vi "Decorate.vi"(10 "Queue":refnum<class "Queue.lvclass">, 11 "TEMPLATE Queue in":refnum<class "TEMPLATE Queue.lvclass">) -> (3 "TEMPLATE Queue out":refnum<class "TEMPLATE Queue.lvclass">)   [LabVIEW 2021, in "_Template.lvlib" / "Templates.lvlib" / "TEMPLATE Queue.lvlib" / "TEMPLATE Queue.lvclass"]
uses:
  TEMPLATE Queue.lvclass
  <vilib>/Nathan Davis/jettl/jettl/Queue/Queue.lvclass
  TEMPLATE Queue.lvclass/TEMPLATE Queue.ctl
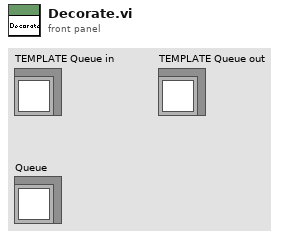
[diagram p1: front panel]
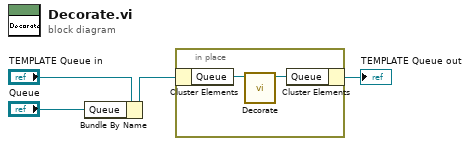
[diagram p0: block diagram]
diagram:
  n1 = Bundle By Name(cluster="TEMPLATE Queue in", "Queue"="Queue") -> (w2:refnum<class "TEMPLATE Queue.lvclass">)
  n2 = in-place {
    n3 = in-place-cluster #1(w2) -> ("Queue"=w6:refnum<class "Queue.lvclass">)
    n4 = call-dynamic "Decorate.vi"("Queue in"=w6) -> ("Queue out"=w5:refnum<class "Queue.lvclass">)  [unwired: 10 in]
    n5 = in-place-cluster #1("Queue"=w5) -> (→"TEMPLATE Queue out":refnum<class "TEMPLATE Queue.lvclass">)
  }
